vi "Create QMH.vi"(8 "error in (no error)":errorcluster) -> (0 "error out":errorcluster, 3 "Queue Message Handler":refnum<queue>)   [LabVIEW 2020, in "QHM.lvlib"]
uses:
  QHM.lvlib
  Type Defs/QMH Cluster.ctl
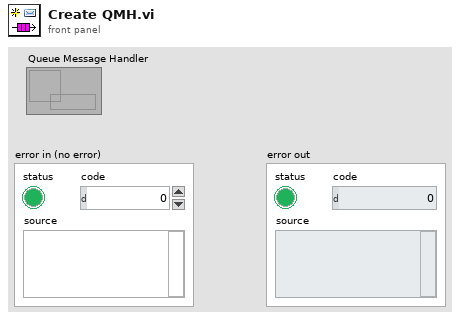
[diagram p1: front panel]
types:
  T1 = typedef "QHM.lvlib/QMH Cluster.ctl" = cluster{"Event":string, "Message":variant}
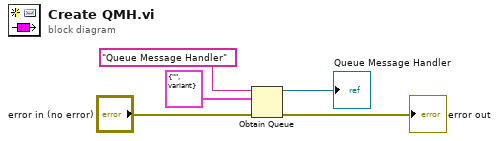
[diagram p0: block diagram]
diagram:
  n1 = Obtain Queue(name (unnamed)="Queue Message Handler", element data type=T1 {"Event"="", "Message"=variant}, error in (no error)="error in (no error)") -> (queue out=→"Queue Message Handler":refnum<queue>, error out=→"error out":errorcluster)  [unwired: 2 in, 1 out]
